vi "Vector Matrix Multiply.vi"(1 "p":i32, 2 "n":i32, 3 "B":sgl[](array[numeric]), 4 "A":sgl[](array[numeric])) -> (0 "C":sgl[](array[numeric]))   [LabVIEW 2020]
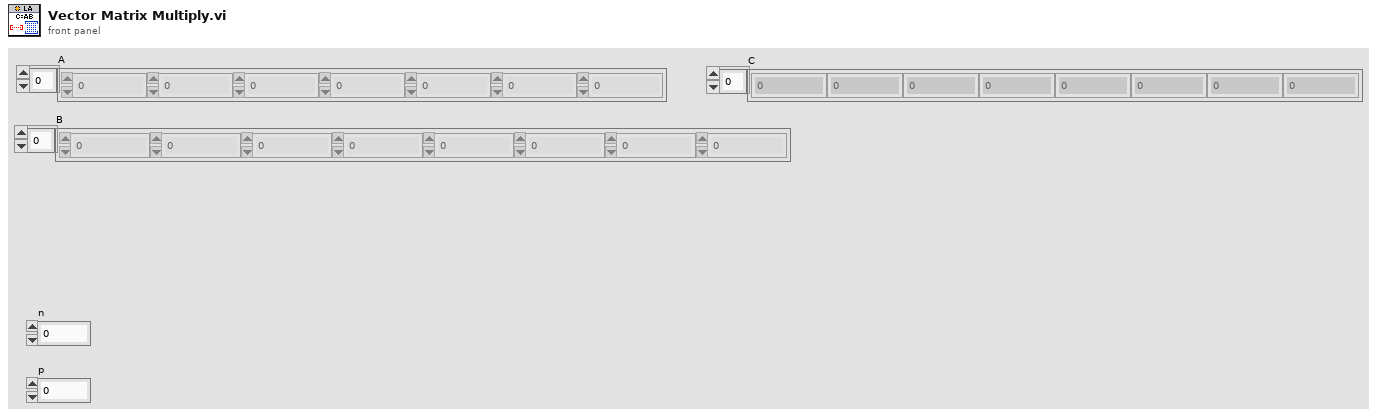
[diagram p1: front panel]
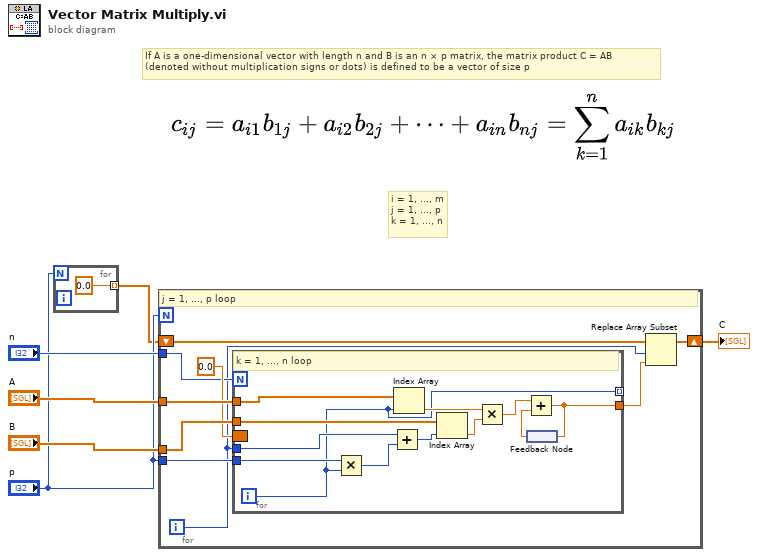
[diagram p0: block diagram]
diagram:
  # "If A is a one-dimensional vector with length n and B is an n × p matrix, the matrix product C = AB \n(denoted without multiplication signs or dots) is defined to be a vector of size p"
  # "i = 1, ..., m\nj = 1, ..., p\nk = 1, ..., n"
  n1 = for {
    N: "p" -> [_]
    tunnel: [sgl 0.0] -> w1 mode=indexing
  }
  n2 = for {
    N: "p" -> [_]
    tunnel: "A" -> [w16]
    tunnel: "B" -> [w15]
    tunnel: "n" -> [w10]
    tunnel: "p" -> [w9]
    shift-right: [w12] -> w4
    shift-left: w1 -> [w13]
    i -> [w8]
    # "j = 1, ..., p loop"
    n3 = for {
      N: w10 -> [_]
      tunnel: w16 -> [w28]
      tunnel: w15 -> [w27]
      tunnel: w8 -> [w21]
      tunnel: [w22] -> w11
      tunnel: w9 -> [w20]
      tunnel: [w17] -> _ mode=indexing
      border: sgl 0.0 -> [_]
      i -> [w17]
      # "k = 1, ..., n loop"
      n4 = Multiply(x=w20, y=w17) -> (x*y=w19:i32)
      n5 = Add(x=w21, y=w19) -> (x+y=w18:i32)
      n6 = Index Array(array=w28, index=w17) -> (element=w26:sgl)
      n7 = Index Array(array=w27, index=w18) -> (element=w25:sgl)
      n8 = Multiply(x=w26, y=w25) -> (x*y=w24:sgl)
      n9 = feedback #1() -> (w23:sgl)
      n10 = Add(x=w24, y=w23) -> (x+y=w22:sgl)
      n11 = feedback-in #1(w22) -> ()
    }
    n12 = Replace Array Subset(array=w13, new element=w11, index=w8) -> (w12:sgl[])
  }
  "C" <- w4
